vi "Read Primary Measurement.vi"(8 "error in (no error)":errorcluster, 11 "VISA resource name":refnum<visa-resource-name>) -> (0 "error out":errorcluster, 1 "Unit":string, 2 "Reading Value":dbl, 3 "VISA resource name out":refnum<visa-resource-name>, 4 "Attribute":string, 5 "State":string)   [LabVIEW 2015, in "Fluke 289.lvlib"]
doc: "Reads primary measurement value."
uses:
  <instrlib>/Fluke 289/Fluke 289.lvlib
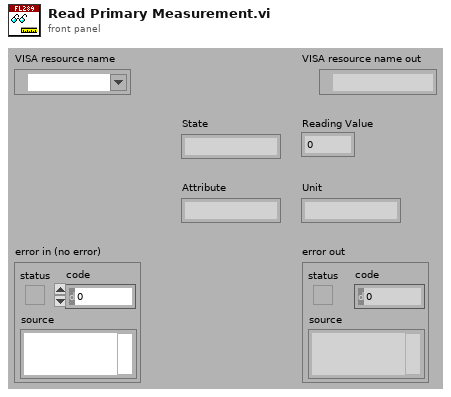
[diagram p1: front panel]
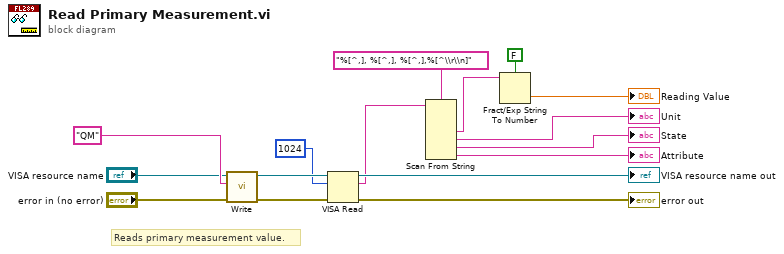
[diagram p0: block diagram]
diagram:
  # "Reads primary measurement value."
  n1 = call <instrlib>:"Write.vi"("error in (no error)"="error in (no error)", "Write Buffer"="QM", "VISA resource name"="VISA resource name") -> ("error out"=w12:errorcluster, "VISA resource name out"=w13:refnum<visa-resource-name>)  [unwired: 7 in]
  n2 = VISA Read(VISA resource name=w13, byte count=u32 1024, error in (no error)=w12) -> (VISA resource name out=→"VISA resource name out":refnum<visa-resource-name>, read buffer=w7:string, error out=→"error out":errorcluster)  [unwired: 1 out]
  n3 = Scan From String(format string="%[^,], %[^,], %[^,],%[^\\r\\n]", input string=w7) -> (output 1=w3:string, output 2=→"Unit":string, output 3=→"State":string, output 4=→"Attribute":string)  [unwired: 6 in, 3 out]
  n4 = Fract/Exp String To Number(use system decimal point (T)=FALSE, string=w3) -> (number=→"Reading Value":dbl)  [unwired: 2 in, 1 out]
